vi "Format ms to timestamp.vi"(11 "Time(ms)":i64=125200) -> (3 "Time Stamp":string)   [LabVIEW 2014, in "Utilities.lvlib"]
uses:
  Utilities.lvlib
panel:
  out "days":i16
  out "milliseconds":i16
  out "seconds":i16
  out "minutes":i16
  out "hours":i16
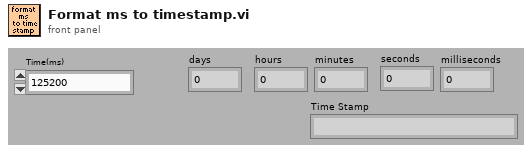
[diagram p1: front panel]
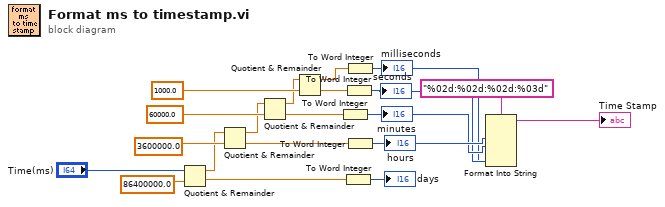
[diagram p0: block diagram]
diagram:
  n1 = Quotient & Remainder(x="Time(ms)", y=86400000.0) -> (x-y*floor(x/y)=w13:dbl, floor(x/y)=w9:dbl)
  n2 = Quotient & Remainder(x=w13, y=3600000.0) -> (x-y*floor(x/y)=w18:dbl, floor(x/y)=w12:dbl)
  n3 = Quotient & Remainder(x=w18, y=60000.0) -> (x-y*floor(x/y)=w16:dbl, floor(x/y)=w11:dbl)
  n4 = Quotient & Remainder(x=w16, y=1000.0) -> (x-y*floor(x/y)=w8:dbl, floor(x/y)=w10:dbl)
  n5 = To Word Integer(number=w11) -> (16bit integer=w5:i16)
  "minutes" <- w5
  n6 = To Word Integer(number=w9) -> (16bit integer=→"days":i16)
  n7 = To Word Integer(number=w10) -> (16bit integer=w4:i16)
  "seconds" <- w4
  n8 = To Word Integer(number=w8) -> (16bit integer=w3:i16)
  "milliseconds" <- w3
  n9 = To Word Integer(number=w12) -> (16bit integer=w6:i16)
  "hours" <- w6
  n10 = Format Into String(format string="%02d:%02d:%02d:%03d", w6, w5, w4, w3) -> (resulting string=→"Time Stamp":string)  [unwired: 2 in, 1 out]
